vi "GenINI_Guess_Type.vi"(8 "error in (no error)":errorcluster, 11 "key value":string) -> (0 "error out":errorcluster, 3 "Guessed type":T1=enum."I32")   [LabVIEW 2009]
uses:
  Typedefs/GenINI_Read_Types.ctl
  <vilib>/regexp/Match Regular Expression.xnode
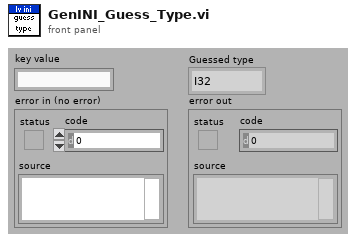
[diagram p1: front panel]
types:
  T1 = typedef "GenINI_Read_Types.ctl" = enum16{"Boolean", "Double", "I32", "Path", "String", "U32"}
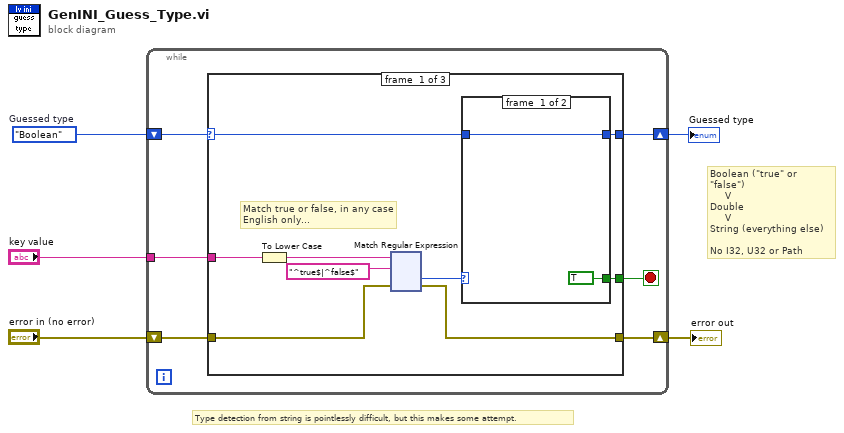
[diagram p0: block diagram]
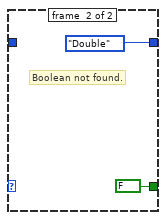
[diagram p2: hidden frame]
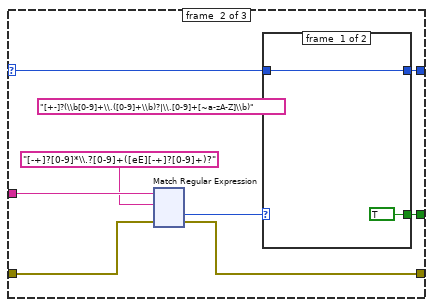
[diagram p3: hidden frame]
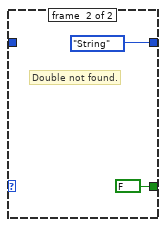
[diagram p4: hidden frame]
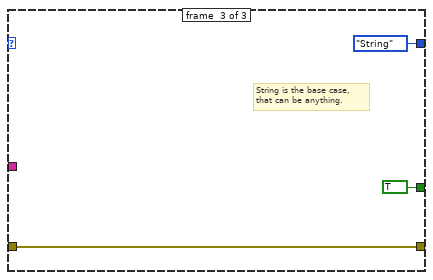
[diagram p5: hidden frame]
diagram:
  w4 = GenINI_Read_Types."Boolean"  # Guessed type
  # "Boolean (\"true\" or \"false\")\n     V\nDouble\n     V\nString (everything else)\n\nNo I32, U32 or Path"
  # "Type detection from string is pointlessly difficult, but this makes some attempt."
  n1 = while {
    tunnel: "key value" -> [w8]
    shift-right: [w10] -> w3
    shift-left: w4 -> [w11]
    shift-right: [w6] -> w1
    shift-left: "error in (no error)" -> [w7]
    stop <- w9 stop-if-true
    n2 = case shown="\"Double\"" w11 {
      selector: w11 -> [w15 w138 _]
      tunnel: [w14 w137 GenINI_Read_Types."String" ("Guessed type")] -> w10
      tunnel: [w20 w139 TRUE] -> w9
      tunnel: w8 -> [w19 w136 _]
      tunnel: w7 -> [w13 w134 w251]
      tunnel: [w12 w133 w251] -> w6
      frame #0 {
        # "Match true or false, in any case\nEnglish only..."
        n3 = To Lower Case(string=w19) -> (all lower case string=w16:string)
        n4 = xnode "Match Regular Expression"("input string"=w16, "regular expression"="^true$|^false$", "error in"=w13) -> ("offset past match"=w17:i32, "error out"=w12:errorcluster)  [unwired: 3 in, 3 out]
        n5 = case shown="-1" w17 {
          tunnel: [TRUE FALSE] -> w20
          tunnel: w15 -> [w22 _]
          tunnel: [w22 GenINI_Read_Types."Double" ("Guessed type")] -> w14
          frame #0 {
          }
          frame #1 {
            # "Boolean not found."
          }
        }
      }
      frame #1 {
        (unwired) "[+-]?(\\b[0-9]+\\.([0-9]+\\b)?|\\.[0-9]+[~a-zA-Z]\\b)" ("regular expression")
        n6 = xnode "Match Regular Expression"("input string"=w136, "regular expression"="[-+]?[0-9]*\\.?[0-9]+([eE][-+]?[0-9]+)?", "error in"=w134) -> ("offset past match"=w135:i32, "error out"=w133:errorcluster)  [unwired: 3 in, 3 out]
        n7 = case shown="-1" w135 {
          tunnel: [TRUE FALSE] -> w139
          tunnel: w138 -> [w248 _]
          tunnel: [w248 GenINI_Read_Types."String" ("Guessed type")] -> w137
          frame #0 {
          }
          frame #1 {
            # "Double not found."
          }
        }
      }
      frame #2 {
        # "String is the base case,\nthat can be anything."
      }
    }
  }
  "Guessed type" <- w3
  "error out" <- w1
